vi "Tabla.vi"(8 "error in (no error)":errorcluster, 10 "Tabla":i32, 11 "UI Actor in":refnum<class "UI Actor.lvclass">) -> (0 "error out":errorcluster, 3 "UI Actor out":refnum<class "UI Actor.lvclass">)   [LabVIEW 2020]
uses:
  UI Actor.lvclass
panel:
  out "Tabla 2":i32
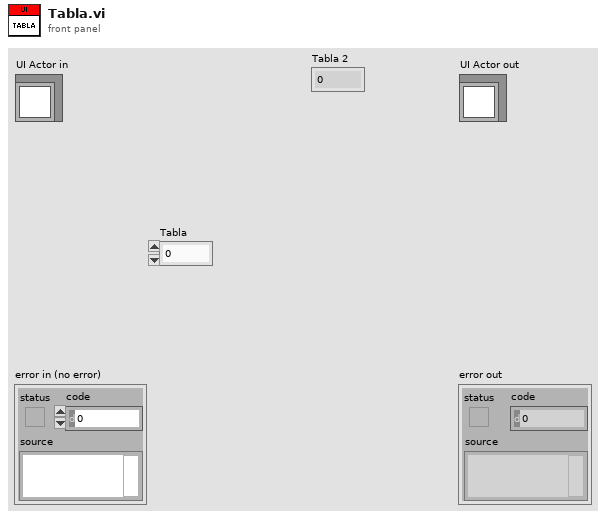
[diagram p1: front panel]
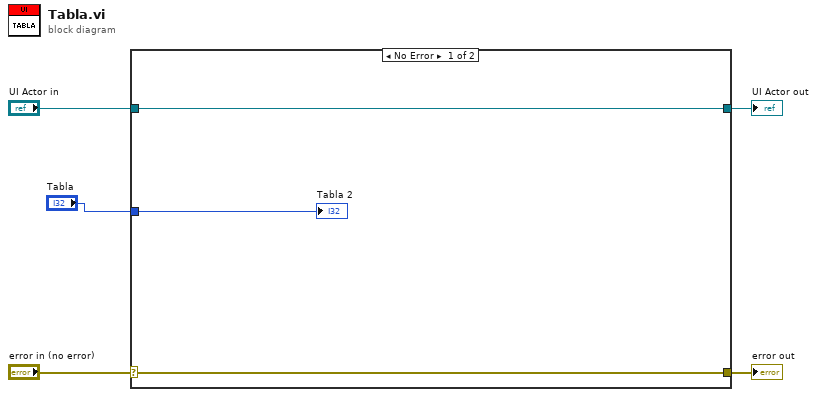
[diagram p0: block diagram]
diagram:
  n1 = case shown="No Error" "error in (no error)" {
    selector: "error in (no error)" -> [w7 w10]
    tunnel: [w7 w10] -> w4
    tunnel: [w8 w9] -> w2
    tunnel: "UI Actor in" -> [w8 w9]
    tunnel: "Tabla" -> [w6 _]
    frame No Error {
      "Tabla 2" <- w6
    }
    frame Error {
    }
  }
  "error out" <- w4
  "UI Actor out" <- w2
